vi "Wait For Error.vi"(8 "error in (no error)":errorcluster, 9 "timeout in ms (0)":i32, 11 "Interface in":refnum<class "Interface.lvclass">) -> (0 "error out":errorcluster, 1 "timed out?":bool, 2 "error":errorcluster, 3 "Interface out":refnum<class "Interface.lvclass">, 4 "# elements":u32)   [LabVIEW 2020, in "DSF Core.lvlib" / "Interface.lvclass"]
uses:
  Interface.lvclass
  Interface.lvclass/Interface.ctl
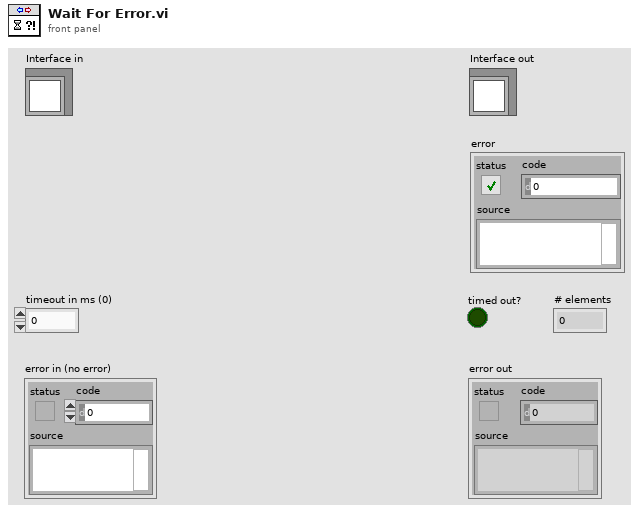
[diagram p1: front panel]
types:
  T1 = enum16{"big-endian, network order", "native, host order", "little-endian"}
  T2 = typedef "DSF Core.lvlib/Framework.lvclass/DSF FIFO Options.ctl" = cluster{"Infinite Timeouts":bool}
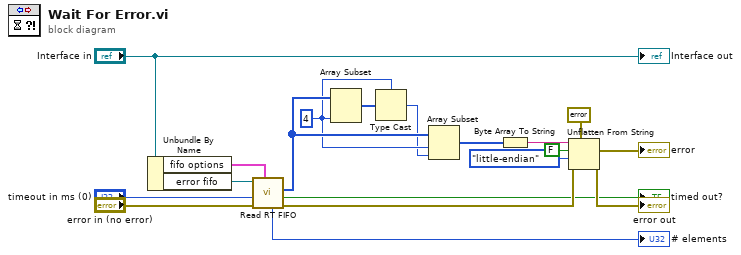
[diagram p0: block diagram]
diagram:
  w8 = 4 ("length")
  n1 = Unbundle By Name("Interface in") -> ("fifo options"=w13:T2, "error fifo"=w14:refnum<k33>)
  n2 = call "Read RT FIFO.vi"("fifo options"=w13, "error in (no error)"="error in (no error)", "timeout in ms (0)"="timeout in ms (0)", "rt fifo in"=w14) -> ("error out"=w18:errorcluster, "empty?"=→"timed out?":bool, "element"=w9:u8[], "# elements"=→"# elements":u32)  [unwired: 3 in, 1 out]
  n3 = Array Subset(array=w9, length=w8) -> (w10:u8[])  [unwired: 1 in]
  n4 = Type Cast(type=w8, x=w10) -> (*(type *) &x=w7:i32)
  n5 = Array Subset(array=w9, index=w8, length=w7) -> (w4:u8[])
  n6 = Byte Array To String(unsigned byte array=w4) -> (string=w3:string)
  n7 = Unflatten From String(type=errorcluster {"status"=FALSE, "code"=0, "source"=""} ("error"), binary string=w3, data includes array or string size? (T)=FALSE, byte order (0:big-endian, network order)=T1."little-endian", error in (no error)=w18) -> (value=→"error":errorcluster, error out=→"error out":errorcluster)  [unwired: 1 out]
  "Interface out" <- "Interface in"
